vi "Should Continue.vi"(8 "error in (no error)":errorcluster, 11 "RepeatingDirector in":refnum<class "RepeatingDirector.lvclass">) -> (0 "error out":errorcluster, 2 "Should Continue":bool, 3 "RepeatingDirector out":refnum<class "RepeatingDirector.lvclass">)   [LabVIEW 2023, in "HAF.lvlib" / "RepeatingDirector.lvclass"]
doc: "Returns False when the Repeat Count equals the Times to Repeat."
uses:
  RepeatingDirector.lvclass
  RepeatingDirector.lvclass/RepeatingDirector.ctl
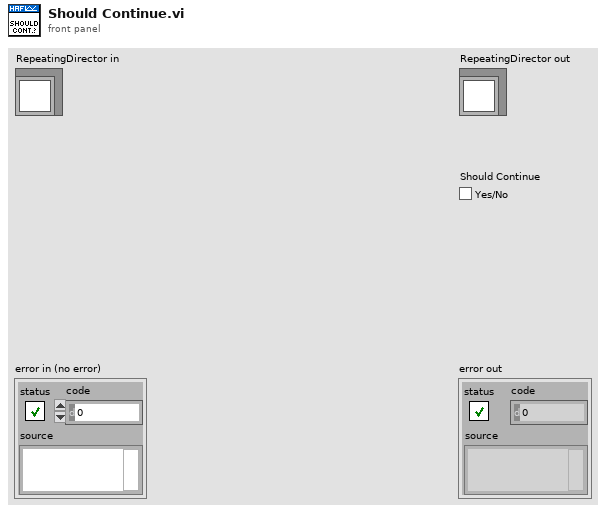
[diagram p1: front panel]
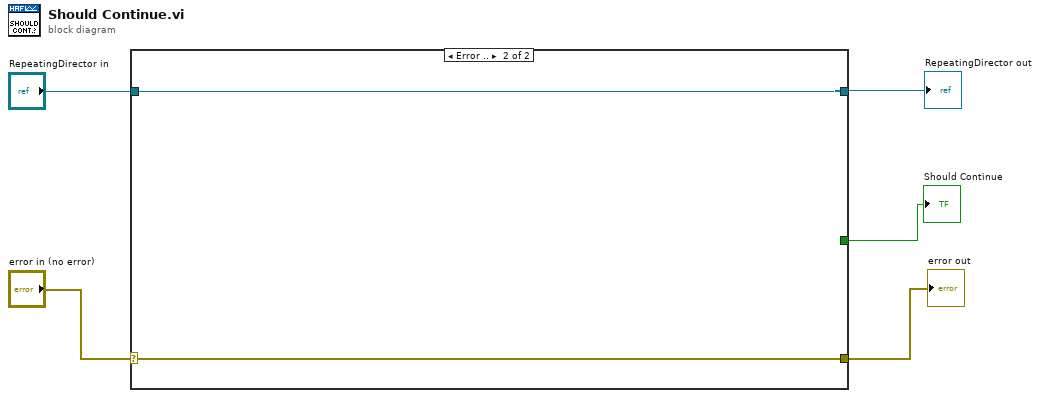
[diagram p0: block diagram]
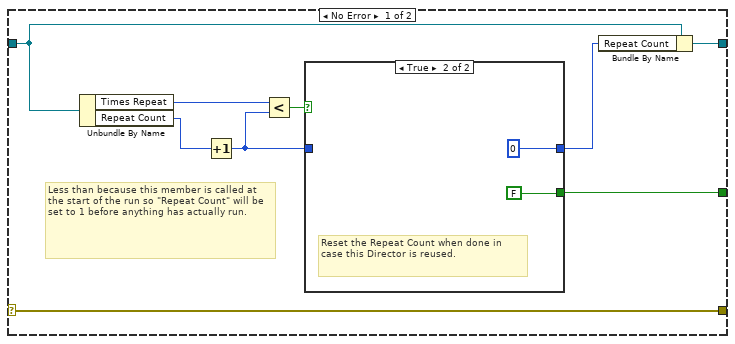
[diagram p2: hidden frame]
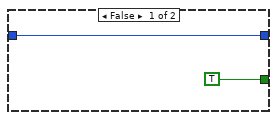
[diagram p3: hidden frame]
diagram:
  n1 = case shown="Error .." "error in (no error)" {
    selector: "error in (no error)" -> [w14 w19]
    tunnel: [w14 w19] -> w4
    tunnel: "RepeatingDirector in" -> [w7 w20]
    tunnel: [w8 w20] -> w2
    tunnel: [w9 _] -> w1
    frame No Error {
      # "Less than because this member is called at the start of the run so \"Repeat Count\" will be set to 1 before anything has actually run."
      n2 = Unbundle By Name(w7) -> ("Times Repeat"=w12:u32, "Repeat Count"=w13:u32)
      n3 = Increment(x=w13) -> (x+1=w10:u32)
      n4 = Less?(x=w12, y=w10) -> (x < y?=w11:bool)
      n5 = case shown="True" w11 {
        tunnel: w10 -> [w16 _]
        tunnel: [w16 u32 0] -> w6
        tunnel: [TRUE FALSE] -> w9
        frame False {
        }
        frame True {
          # "Reset the Repeat Count when done in case this Director is reused."
        }
      }
      n6 = Bundle By Name(cluster=w7, "Repeat Count"=w6) -> (w8:refnum<class "RepeatingDirector.lvclass">)
    }
    frame Error {
    }
  }
  "error out" <- w4
  "RepeatingDirector out" <- w2
  "Should Continue" <- w1
